vi "Control - Generic - Turbo Bypass Valve Host.vi"() -> ()   [LabVIEW 2015, in "ECS-Host.lvlib"]
uses:
  ECS-Host.lvlib
panel:
  in  "DiffP_Thresh":sgl caption="[kPa]"
  out "DiffP":sgl caption="[kPa]"
  in  "OnPsn":sgl caption="[%Open]"
  in  "OffPsn":sgl caption="[%Open]"
  out "TurboBPVPsn_Des":sgl caption="[%Open]"
  out "TurboBPVPsn_Calc":sgl caption="[%Open]"
  in  "TurboBPVPsn_ManE":bool caption="ManualWGSetpointEnable"
  in  "TurboBPVPsn_Man":sgl caption="[%Open]"
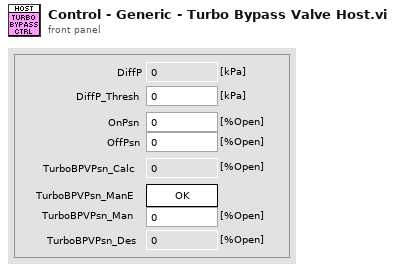
[diagram p1: front panel]
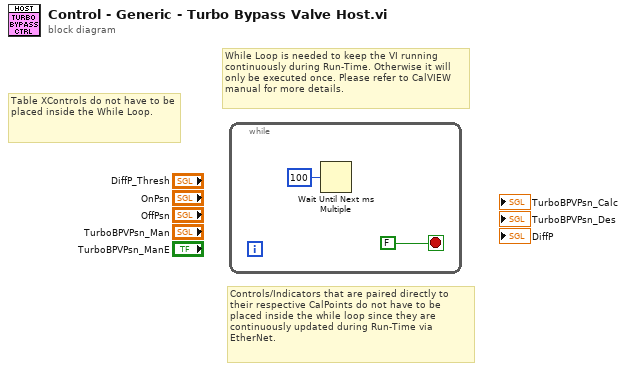
[diagram p0: block diagram]
diagram:
  # "Table XControls do not have to be placed inside the While Loop."
  # "While Loop is needed to keep the VI running\ncontinuously during Run-Time. Otherwise it will only be executed once. Please refer to CalVIEW manual for more details."
  # "Controls/Indicators that are paired directly to their respective CalPoints do not have to be placed inside the while loop since they are continuously updated during Run-Time via EtherNet."
  n1 = while {
    stop <- FALSE stop-if-true
    n2 = Wait Until Next ms Multiple(millisecond multiple=u32 100) -> ()  [unwired: 1 out]
  }
